vi "Recovery PN.vi"(8 "error in (no error)":errorcluster caption="entrée d'erreur (pas d'erreur)", 11 "Firebase Benches en entrée":refnum<class "Firebase Recovery_SN.lvclass">) -> (0 "error out":errorcluster caption="sortie d'erreur", 3 "Firebase Benches en sortie":refnum<class "Firebase Recovery_SN.lvclass">)   [LabVIEW 2020, in "Library Instrument & Equipement.lvlib" / "Library FireBase.lvlib" / "Firebase Recovery_SN.lvclass"]
doc: "Returns data according to Value_To_Find on Collection_to_find Use Nb_To_Read to determine the number to read\nPlease initialise the following values before use the VI\n - Name BDD\n - Value to find\n - API Key\n - Field Filter\n - Field Order\n - Collection_to_find\n\nIf there is no Field order -> Field Order=Field Filter"
uses:
  Firebase Recovery_SN.lvclass
  C:/Users/ngarcin/OneDrive - Altyor/Standard TB/Class/Firebase/Source/Firebase Driver/Firebase Driver.lvclass
  Firebase Recovery_SN.lvclass/Firebase Recovery_SN.ctl
  JSON API/JSON Value/Set from JSON string.vi
  JSON API/JSON Value/JSON Value.lvclass
  JSON API/Variant JSON/Variant JSON.lvlib
  JSON API/Get Polymorphic/JSON GetSet.lvlib
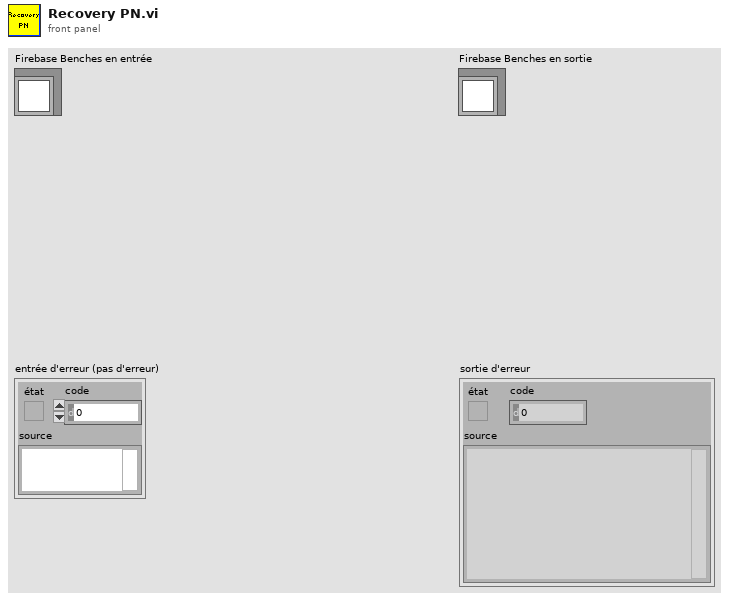
[diagram p1: front panel]
types:
  T1 = enum16{"Get Document", "Delete Document", "Get Format SN", "Add in All ready use"}[]
  T2 = cluster{"name":string, "fields":cluster{"Value":cluster{"stringValue":string}}}[]
  T3 = cluster{"name":string, "fields":cluster{"Value":cluster{"stringValue":string}}}
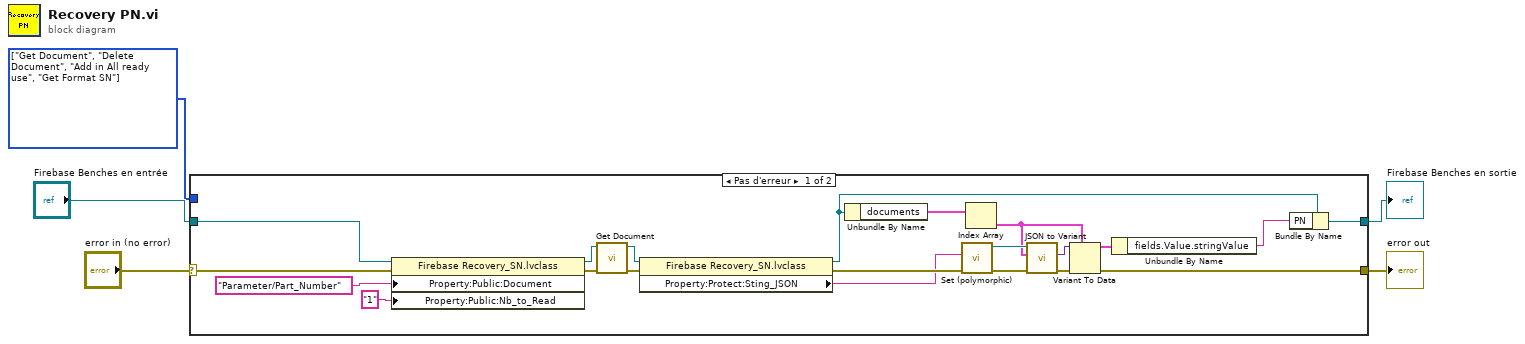
[diagram p0: block diagram]
diagram:
  w1 = T1 [enum."Get Document", enum."Delete Document", enum."Add in All ready use", enum."Get Format SN"] items=["Get Document", "Delete Document", "Get Format SN", "Add in All ready use"]
  n1 = case shown="Pas d'erreur" "error in (no error)" {
    selector: "error in (no error)" -> [w25 w28]
    tunnel: "Firebase Benches en entrée" -> [w26 w27]
    tunnel: [w23 w28] -> w4
    tunnel: [w24 w27] -> w3
    tunnel: w1 -> [_ _]
    frame No Error {
      n2 = property class="Firebase Recovery_SN.lvclass"(reference=w26, error in=w25, "Property:Public:Document"="Parameter/Part_Number" ("Collection_to_find"), "Property:Public:Nb_to_Read"="1" ("Nb_to_Read")) -> (reference out=w20:refnum<class "Firebase Recovery_SN.lvclass">, error out=w21:errorcluster)
      n3 = call-dynamic "Get Document.vi"("error in (no error)"=w21, "Firebase (Default) en entrée"=w20) -> ("error out"=w12:errorcluster, "Firebase (Default) en sortie"=w11:refnum<class "Firebase Recovery_SN.lvclass">)  [unwired: 8 in]
      n4 = property class="Firebase Recovery_SN.lvclass"(reference=w11, error in=w12) -> (reference out=w10:refnum<class "Firebase Recovery_SN.lvclass">, error out=w17:errorcluster, "Property:Protect:Sting_JSON"=w16:string)
      n5 = Unbundle By Name(w10) -> ("documents"=w8:T2)
      n6 = call-poly "Set (polymorphic).vi"("error in (no error)"=w17, "JSON stream"=w16) -> ("error out"=w15:errorcluster, "JSON Value out"=w13:refnum<class "JSON Value.lvclass">)  [unwired: 7 in, 1 out]
      n7 = Index Array(array=w8) -> (element=w6:T3)  [unwired: 1 in]
      n8 = call "JSON to Variant.vi"("error in (no error)"=w15, "Variant (Data Type)"=w6, "JSON Value"=w13) -> ("error out"=w14:errorcluster, "Variant out"=w18:variant)  [unwired: 7 in]
      n9 = Variant To Data(error in=w14, type=w6, Variant=w18) -> (data=w7:T3, error out=w23:errorcluster)
      n10 = Unbundle By Name(w7) -> ("fields.Value.stringValue"=w9:string)
      n11 = Bundle By Name(cluster=w10, "PN"=w9) -> (w24:refnum<class "Firebase Recovery_SN.lvclass">)
    }
    frame Error {
    }
  }
  "error out" <- w4
  "Firebase Benches en sortie" <- w3
